vi "Stop Log.vi"(8 "error in (no error)":errorcluster, 11 "DemoApp in":refnum<class "DemoApp.lvclass">) -> (0 "error out":errorcluster, 3 "DemoApp out":refnum<class "DemoApp.lvclass">)   [LabVIEW 2020, in "VolatusDemo.lvlib" / "DemoApp.lvclass"]
uses:
  DemoApp.lvclass
  DemoApp.lvclass/DemoApp.ctl
  VolatusDataLogger/LoggingAPI/LoggingAPI.lvclass
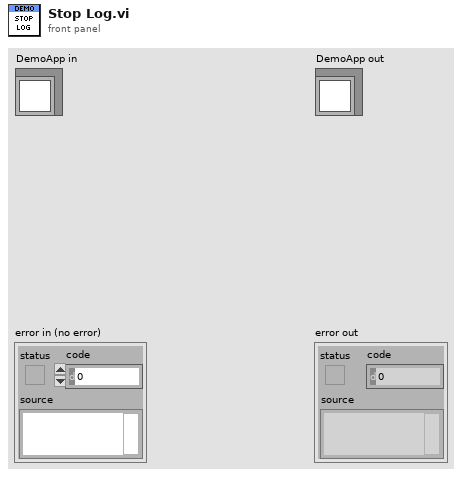
[diagram p1: front panel]
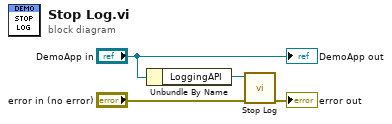
[diagram p0: block diagram]
diagram:
  n1 = Unbundle By Name("DemoApp in") -> ("LoggingAPI"=w3:refnum<class "LoggingAPI.lvclass">)
  n2 = call "Stop Log.vi"("error in (no error)"="error in (no error)", "LoggingAPI in"=w3) -> ("error out"=→"error out":errorcluster)  [unwired: 8 in, 1 out]
  "DemoApp out" <- "DemoApp in"
